vi "BrakingState.vi"(6 "Actual Start [i]":i64, 8 "error in (no error)":errorcluster, 9 "Cluster in":T2, 10 "Enum in":T1, 11 "Velocity":dbl) -> (0 "error out":errorcluster, 2 "Cluster":T2, 3 "Enum":T1)   [LabVIEW 2018]
uses:
  Type_Def/Type_Def Actuator Controls.ctl
  Type_Def/Type_Def ControlState.ctl
panel:
  out "x+1":i16
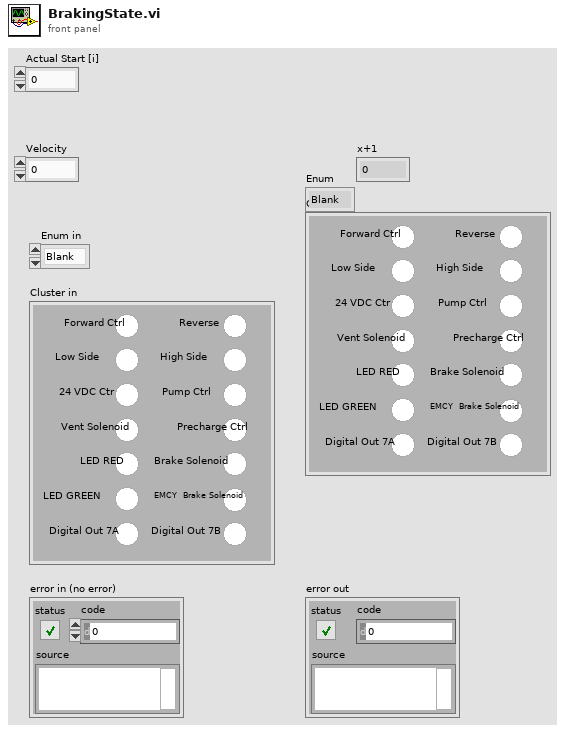
[diagram p1: front panel]
types:
  T1 = typedef "Type_Def ControlState.ctl" = enum16{"Blank", "Systems Check", "Idle", "Ready", "Pushing", "CrawlingPrecharge", "Braking", "Fault", "Boot Up", "Crawling", "Shutdown", "Service Push", "Service Wait", "Vent", "Precharge"}
  T2 = typedef "Type_Def Actuator Controls.ctl" = cluster{"Reverse ":bool, "Precharge Ctrl":bool, "Pump Ctrl":bool, "24 VDC Ctr":bool, "Vent Solenoid":bool, "Brake Solenoid":bool, "EMCY  Brake Solenoid":bool, "Digital Out 7B ":bool, "Forward Ctrl":bool, " Low Side":bool, "High Side":bool, "LED RED":bool, "LED GREEN":bool, " Digital Out 7A":bool}
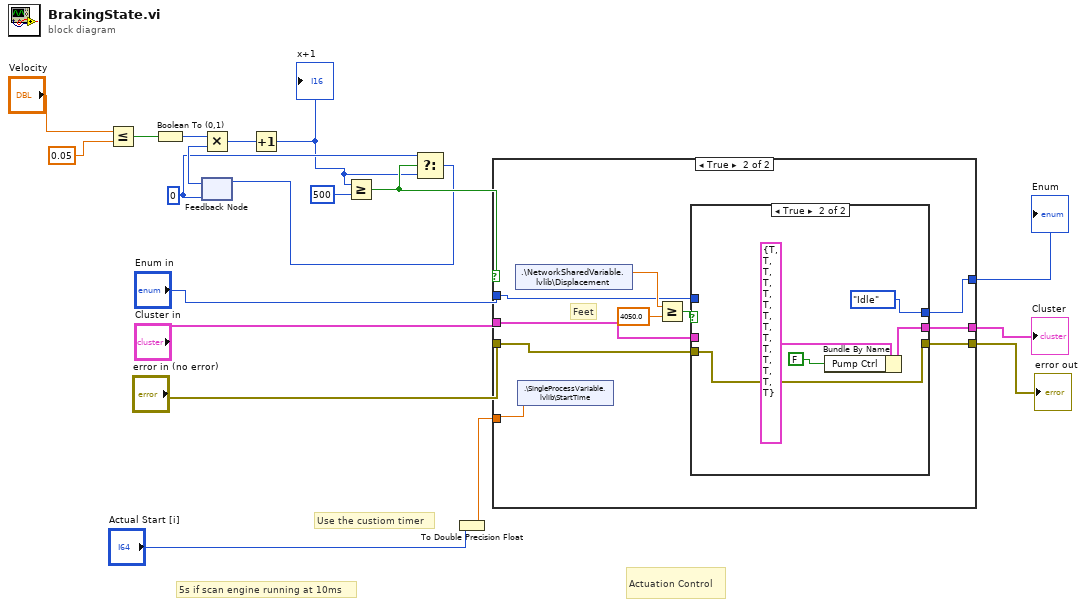
[diagram p0: block diagram]
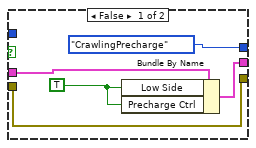
[diagram p3: hidden frame]
diagram:
  w4 = i16 0
  # "5s if scan engine running at 10ms"
  # "Use the custiom timer"
  # "Actuation Control"
  n1 = Less Or Equal?(x="Velocity", y=0.05) -> (x <= y?=w15:bool)
  n2 = Boolean To (0,1)(Boolean=w15) -> (0, 1=w16:i16)
  n3 = feedback #1(w4) -> (w19:i16)
  n4 = Multiply(x=w16, y=w19) -> (x*y=w17:i16)
  n5 = Increment(x=w17) -> (x+1=w2:i16)
  "x+1" <- w2
  n6 = Greater Or Equal?(x=w2, y=i16 500) -> (x >= y?=w3:bool)
  n7 = Select(t=w4, s=w3, f=w2) -> (s? t:f=w1:i16)
  n8 = feedback-in #1(w1) -> ()
  n9 = To Double Precision Float(number="Actual Start [i]") -> (double precision float=w5:dbl)
  n10 = case shown="True" w3 {
    tunnel: "Enum in" -> [w22 w24]
    tunnel: [w22 w25] -> w9
    tunnel: "Cluster in" -> [w21 w26]
    tunnel: [w21 w27] -> w11
    tunnel: [w20 w29] -> w12
    tunnel: "error in (no error)" -> [w20 w28]
    tunnel: w5 -> [_ w23]
    frame False {
      # "Pass the value for the next state through"
    }
    frame True {
      # "Feet"
      n11 = shared-variable ".\\NetworkSharedVariable.lvlib\\Displacement"() -> (w32:dbl)  [unwired: 1 in, 1 out]
      n12 = shared-variable ".\\SingleProcessVariable.lvlib\\StartTime"(w23) -> ()  [unwired: 1 in, 1 out]
      n13 = Greater Or Equal?(x=w32, y=4050.0) -> (x >= y?=w30:bool)
      n14 = case shown="True" w30 {
        tunnel: [w36 w39] -> w29
        tunnel: w28 -> [w36 w39]
        tunnel: [w34 w40] -> w27
        tunnel: w26 -> [w35 _]
        tunnel: [Type_Def_ControlState."CrawlingPrecharge" Type_Def_ControlState."Idle"] -> w25
        tunnel: w24 -> [_ _]
        frame False {
          w33 = TRUE ("Digital Out 5")
          n15 = Bundle By Name(cluster=w35, "Low Side"=w33, "Precharge Ctrl"=w33) -> (w34:T2)
        }
        frame True {
          n16 = Bundle By Name(cluster=T2 {"Reverse "=TRUE, "Precharge Ctrl"=TRUE, "Pump Ctrl"=TRUE, "24 VDC Ctr"=TRUE, "Vent Solenoid"=TRUE, "Brake Solenoid"=TRUE, "EMCY  Brake Solenoid"=TRUE, "Digital Out 7B "=TRUE, "Forward Ctrl"=TRUE, " Low Side"=TRUE, "High Side"=TRUE, "LED RED"=TRUE, "LED GREEN"=TRUE, " Digital Out 7A"=TRUE}, "Pump Ctrl"=FALSE ("Digital Out 5")) -> (w40:T2)
        }
      }
    }
  }
  "error out" <- w12
  "Cluster" <- w11
  "Enum" <- w9
